vi "NewBoard.vi"() -> (0 "error out":errorcluster)   [LabVIEW 2014]
uses:
  <vilib>/Instr/_visa.llb/VISA Configure Serial Port (Instr).vi
panel:
  in  "stop":bool
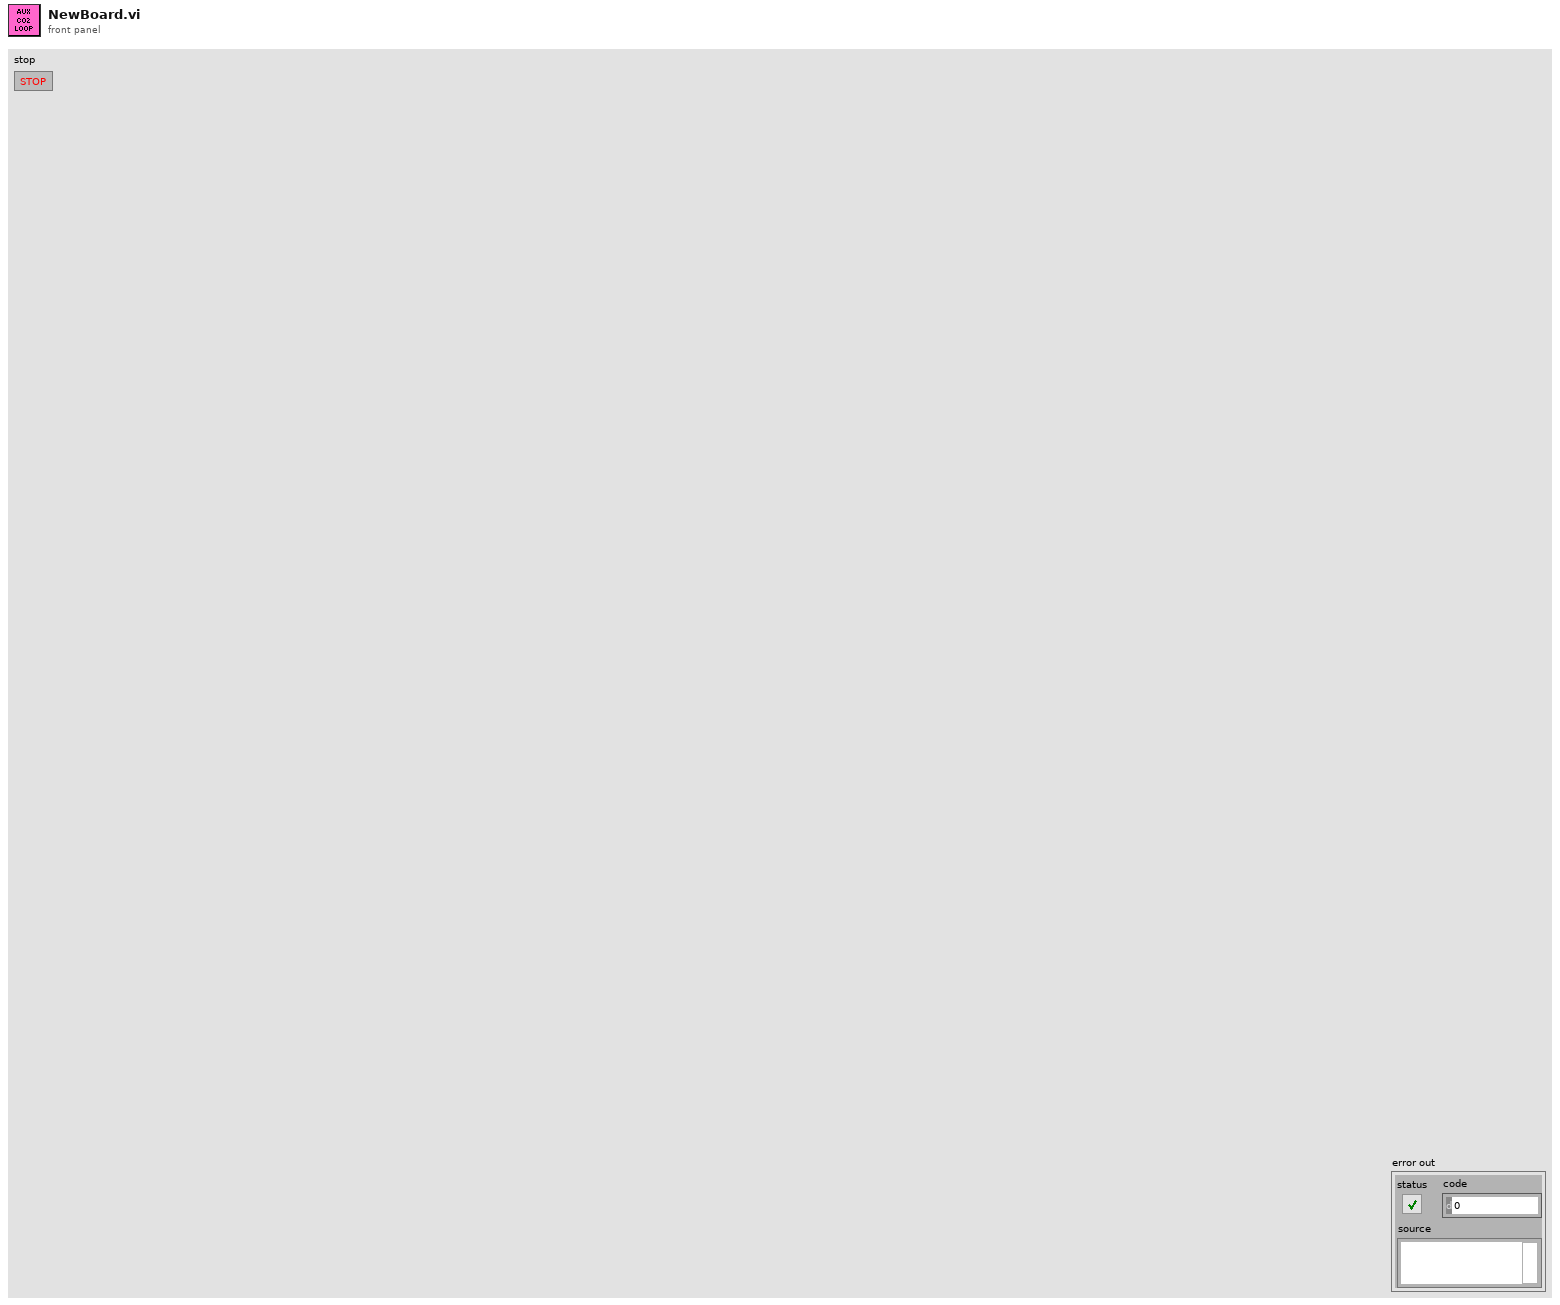
[diagram p1: front panel]
types:
  T1 = typedef "Aux CO2 Diags.ctl" = cluster{"Port":refnum<visa-resource-name>, "Source":T2, "Active":bool, "Baro Pressure":u16, "SerialRxBuffer":string, "Raw CO2 (Torr)":sgl, "bytes read":i16, "Status":u8[], "Status Message":enum16{"", "Sensor Over Temp", "Sensor Faulty", "Set BaroP", "Capno in Sleep Mode", "Zero In Progress", "Sensor Warm Up", "Check Sampling Line", "Zero Required", "CO2 Out Of Range", "Check Airway Adapter", "LoFlo Not Connected"}}
  T2 = typedef "Aux CO2 Selector.ctl" = u16
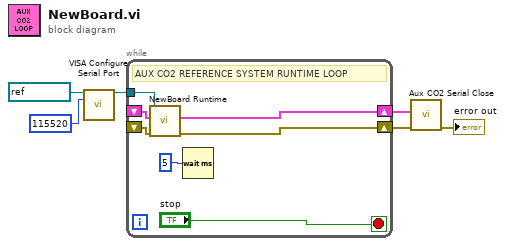
[diagram p0: block diagram]
diagram:
  n1 = call-poly "VISA Configure Serial Port"("VISA resource name"=refnum<visa-resource-name> "COM7" ("Serial Port.VISA resource name"), "baud rate (9600)"=u32 115520 ("Serial Port.baud rate")) -> ("VISA resource name out"=w1:refnum<visa-resource-name>)  [unwired: 12 in, 1 out]
  n2 = while {
    shift-right: [w10] -> w5
    shift-left: _ -> [w11]
    shift-right: [w9] -> w6
    shift-left: _ -> [w12]
    tunnel: w1 -> [w7]
    stop <- "stop" stop-if-true
    # "AUX CO2 REFERENCE SYSTEM RUNTIME LOOP"
    n3 = call "NewBoard Runtime.vi"("error in (no error)"=w12, "Capno Data In"=w11, "reference"=w7) -> ("Error Out"=w9:errorcluster, "Capno Data Out"=w10:T1)  [unwired: 5 in, 2 out]
    n4 = Wait (ms)(milliseconds to wait=u32 5) -> ()  [unwired: 1 out]
  }
  n5 = call "Aux CO2 Serial Close.vi"("error in"=w6, "Capno Data In"=w5) -> ("error out"=→"error out":errorcluster)  [unwired: 7 in, 2 out]
